vi "RTD_volts-to-temp-v2-RTD-830.vi"(11 "RTD Volts":dbl) -> (3 "Temp":dbl)   [LabVIEW 2012]
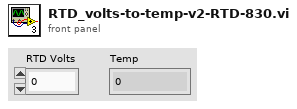
[diagram p1: front panel]
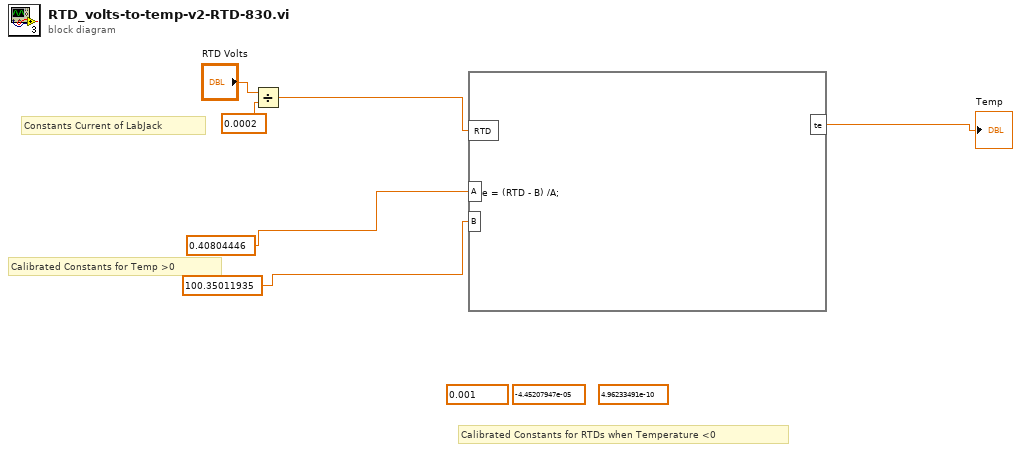
[diagram p0: block diagram]
diagram:
  (unwired) 0.001 ("y")
  (unwired) -4.45207947e-05 ("y")
  (unwired) 4.96233491e-10 ("y")
  # "Constants Current of LabJack"
  # "Calibrated Constants for Temp >0"
  # "Calibrated Constants for RTDs when Temperature <0"
  n1 = Divide(x="RTD Volts", y=0.0002) -> (x/y=w2:dbl)
  n2 = formula code="te = (RTD - B) /A;" ("DEFAULT RTD CONVERSION")("RTD"=w2, "A"=0.40804446 ("y"), "B"=100.35011935 ("y")) -> ("te"=→"Temp":dbl)
